vi "checkBeginEnemyPossesionAtOurField.vi"(8 "error in (no error)":errorcluster, 10 "Game":refnum<class "Game.lvclass">, 11 "EnemyPossessionAtOurFieldPlay in":refnum<class "EnemyPossessionAtOurFieldPlay.lvclass">) -> (0 "error out":errorcluster, 2 "Begin?":bool, 3 "EnemyPossessionAtOurFieldPlay out":refnum<class "EnemyPossessionAtOurFieldPlay.lvclass">)   [LabVIEW 2024, in "EnemyPossessionAtOurFieldPlay.lvclass"]
uses:
  EnemyPossessionAtOurFieldPlay.lvclass
  Game_class/Game.lvclass
  Team_class/OffensivePlay.ctl
  Referee_class/command_interpreted.ctl
  Events_class/Possession.ctl
  Game_class/Game.lvclass/Game.ctl
  Referee_class/Referee.lvclass/Referee.ctl
  Team_class/Team.lvclass/Team.ctl
  Parameters_class/Parameters.lvclass/Parameters.ctl
  Events_class/Events.lvclass/Events.ctl
  Game_class/Read Referee.vi
  Game_class/Read EventsRef.vi
  Game_class/Read OffensiveTeam.vi
  Game_class/Read Parameters.lvclass.vi
  Parameters_class/Read AttakingOurselves.vi
  Team_class/Read OffensivePlay.vi
  Events_class/Read id_touch.vi
  Events_class/Read touch.vi
  Referee_class/Read command_interpreted.vi
  Ally_class/Ally.lvclass
  C:/Users/as119/OneDrive/Documentos/roboIME/SSL_AI/Team_class/Team.lvclass
  Referee_class/Referee.lvclass
  Events_class/Events.lvclass
  Parameters_class/Parameters.lvclass
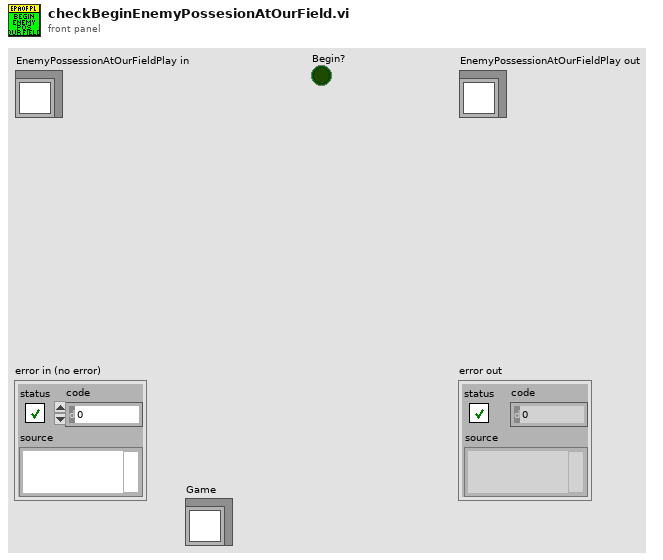
[diagram p1: front panel]
types:
  T1 = typedef "Events.lvclass/Possession.ctl" = enum16{"OurPossession", "TheirPossession", "Contended", "Loose"}
  T2 = typedef "OffensivePlay.ctl" = enum16{"5RobotsPassGamePlay", "5PreparePassGame", "5RobotsKeeperGame", "KeeperPassToStriker", "5RobotsNormalGamePlay", "PrepareKeeperPass", "ACBPass", "ABCPass", "PrepareTriplePass", "TableWithStriker", "TableWith2ndStrikerPlay", "PrepareDoublePass", "PrepareRollToPass", "SimplePass", "PreparePass", "PassToStriker", "BallOutOfField", "PassTo2ndStriker", "StopOffensive", "Prepare Penalty Enemy", "EnemyPossessionAtEnemyField", "EnemyPossesionAtOurField", "TestPlay", "PreparePenaltyAlly", "KickPenaltyAlly", "PrepareKickoffAlly", "PrepareKickoffEnemy", "IndirectEnemy", "DirectEnemy", "PreparePassInGame1", "NormalGame", "DirectKick", "Pass", "Halt", "Timeout", "PassPlay", "PenaltyEnemy"}
  T3 = typedef "command_interpreted.ctl" = enum16{"Goal Ally", "Goal Enemy", "Ball Placement Enemy", "Ball Placement Ally", "Normal Half Time", "Extra Time  Break", "Extra Half Time", "None", "Post Game", "PKA Normal Start", "Prepare Kickoff Ally", "PKE Normal Start", "Prepare Kickoff Enemy", "Force Start", "Halt", "Timeout", "Prepare Penalty Ally", "Prepare Penalty Enemy", "PPA NormalStart", "PPE Normal Start", "Indirect Free Ally", "Direct Free Enemy", "Direct Free Ally", "Indirect Free Enemy", "Stop"}
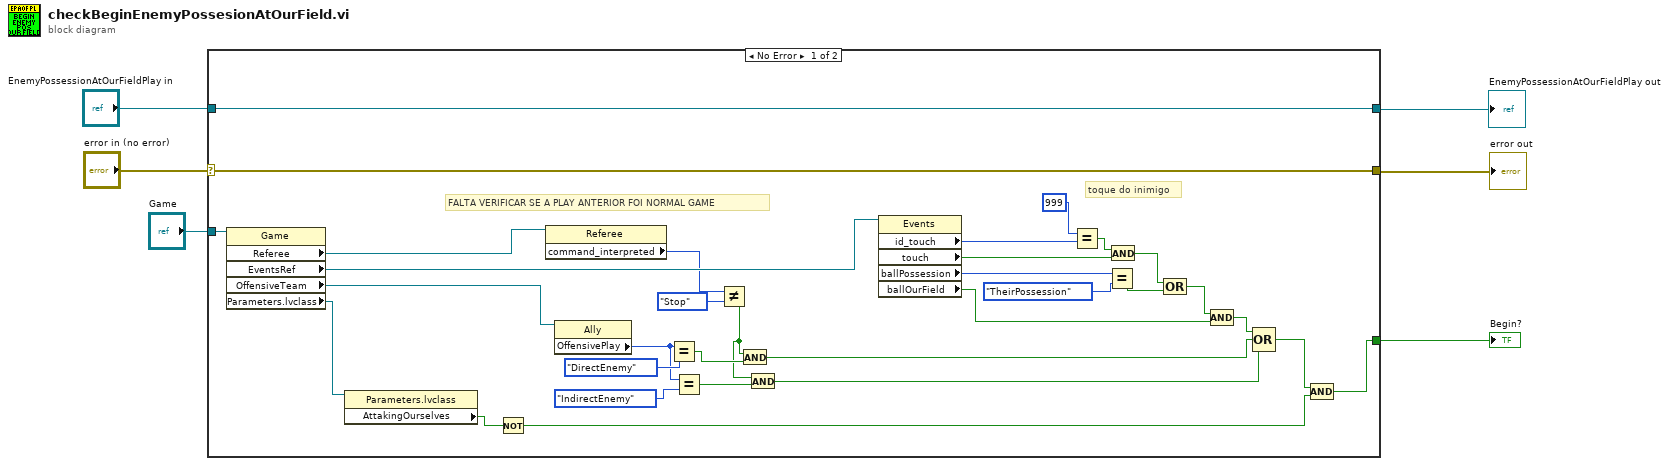
[diagram p0: block diagram]
diagram:
  n1 = case shown="No Error" "error in (no error)" {
    selector: "error in (no error)" -> [w37 w40]
    tunnel: [w37 w40] -> w5
    tunnel: [w38 w39] -> w3
    tunnel: "EnemyPossessionAtOurFieldPlay in" -> [w38 w39]
    tunnel: "Game" -> [w35 _]
    tunnel: [w7 _] -> w1
    frame No Error {
      # "toque do inimigo"
      # "FALTA VERIFICAR SE A PLAY ANTERIOR FOI NORMAL GAME"
      n2 = property class="Game"(reference=w35) -> ("Referee"=w32:refnum<class "Referee.lvclass">, "EventsRef"=w36:refnum<class "Events.lvclass">, "OffensiveTeam"=w12:refnum<class "Ally.lvclass">, "Parameters.lvclass"=w11:refnum<class "Parameters.lvclass">)  [unwired: 1 in, 2 out]
      n3 = property class="Parameters.lvclass"(reference=w11) -> ("AttakingOurselves"=w10:bool)  [unwired: 1 in, 2 out]
      n4 = Not(x=w10) -> (.not. x?=w9:bool)
      n5 = property class="Referee"(reference=w32) -> ("command_interpreted"=w31:T3)  [unwired: 1 in, 2 out]
      n6 = property class="Ally"(reference=w12) -> ("OffensivePlay"=w24:T2)  [unwired: 1 in, 2 out]
      n7 = Equal?(x=w24, y=OffensivePlay."DirectEnemy") -> (x = y?=w33:bool)
      n8 = Equal?(x=w24, y=OffensivePlay."IndirectEnemy") -> (x = y?=w23:bool)
      n9 = Not Equal?(x=w31, y=command_interpreted."Stop") -> (x != y?=w22:bool)
      n10 = And(x=w22, y=w33) -> (x .and. y?=w14:bool)
      n11 = And(x=w22, y=w23) -> (x .and. y?=w13:bool)
      n12 = property class="Events"(reference=w36) -> ("id_touch"=w28:i32, "touch"=w29:bool, "ballPossession"=w21:T1, "ballOurField"=w16:bool)  [unwired: 1 in, 2 out]
      n13 = Equal?(x=999, y=w28) -> (x = y?=w26:bool)
      n14 = Equal?(x=w21, y=Possession."TheirPossession") -> (x = y?=w18:bool)
      n15 = And(x=w26, y=w29) -> (x .and. y?=w19:bool)
      n16 = Compound Arithmetic op=OR(w19, w18) -> (w17:bool)
      n17 = Compound Arithmetic op=AND(w17, w16) -> (w15:bool)
      n18 = Compound Arithmetic op=OR(w15, w14, w13) -> (w8:bool)
      n19 = Compound Arithmetic op=AND(w8, w9) -> (w7:bool)
    }
    frame Error {
    }
  }
  "error out" <- w5
  "EnemyPossessionAtOurFieldPlay out" <- w3
  "Begin?" <- w1
